vi "Get Picture.vi"(8 "error in (no error)":errorcluster, 11 "Device in":refnum<class "Device.lvclass">) -> (0 "error out":errorcluster, 2 "Picture":picture, 3 "Device out":refnum<class "Device.lvclass">)   [LabVIEW 2020, in "PicoG-App.lvlib" / "Device.lvclass"]
uses:
  Device.lvclass
  Builds/picoG/ppl/PicoG-Core.lvlibp/PicoG-Processor/PicoG-Core/PlatformManager/PlatformManager.lvclass
  Builds/picoG/ppl/PicoG-Core.lvlibp/PicoG-Processor/PicoG-Core/Platform/Platform.lvclass
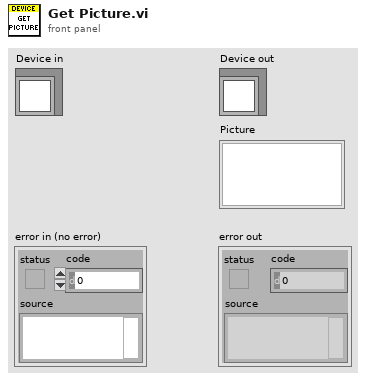
[diagram p1: front panel]
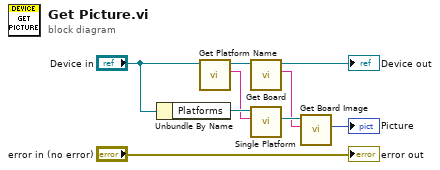
[diagram p0: block diagram]
diagram:
  n1 = Unbundle By Name("Device in") -> ("Platforms"=w7:refnum<class "PlatformManager.lvclass">)
  n2 = call "Get Platform Name.vi"("Device in"="Device in") -> ("Platform"=w6:string, "Device out"=w4:refnum<class "Device.lvclass">)  [unwired: 8 in, 1 out]
  n3 = call "Get Board.vi"("Device in"=w4) -> ("Board"=w3:string, "Device out"=→"Device out":refnum<class "Device.lvclass">)  [unwired: 8 in, 1 out]
  n4 = call "Single Platform.vi"("Platform Name"=w6, "PlatformManager in"=w7) -> ("Platform"=w5:refnum<class "Platform.lvclass">)  [unwired: 7 in, 2 out]
  n5 = call-dynamic "Get Board Image.vi"("Board"=w3, "Platform in"=w5) -> ("Board Image"=→"Picture":picture)  [unwired: 7 in, 2 out]
  "error out" <- "error in (no error)"
